vi "ZCR_IN_SIN_0_finder_temp.vi"(10 "Noise amplitude":dbl format="%.2p", 11 "ZCR IN":waveform(dbl)[](graph)) -> (3 "OFF SIN":i32[](array[numeric]))   [LabVIEW 2020, in "Library Commun.lvlib" / "Nodon_ZCR.lvclass"]
uses:
  Nodon_ZCR.lvclass
  <vilib>/Utility/miscctls.llb/LVRangeTypeDef.ctl
  Nodon_ZCR.lvclass/Nodon_ZCR.ctl
  <vilib>/measure/NI_MABase.lvlib
panel:
  out "Waveform Graph 3":waveform(dbl)[](graph)
  in  "Point 2":i32
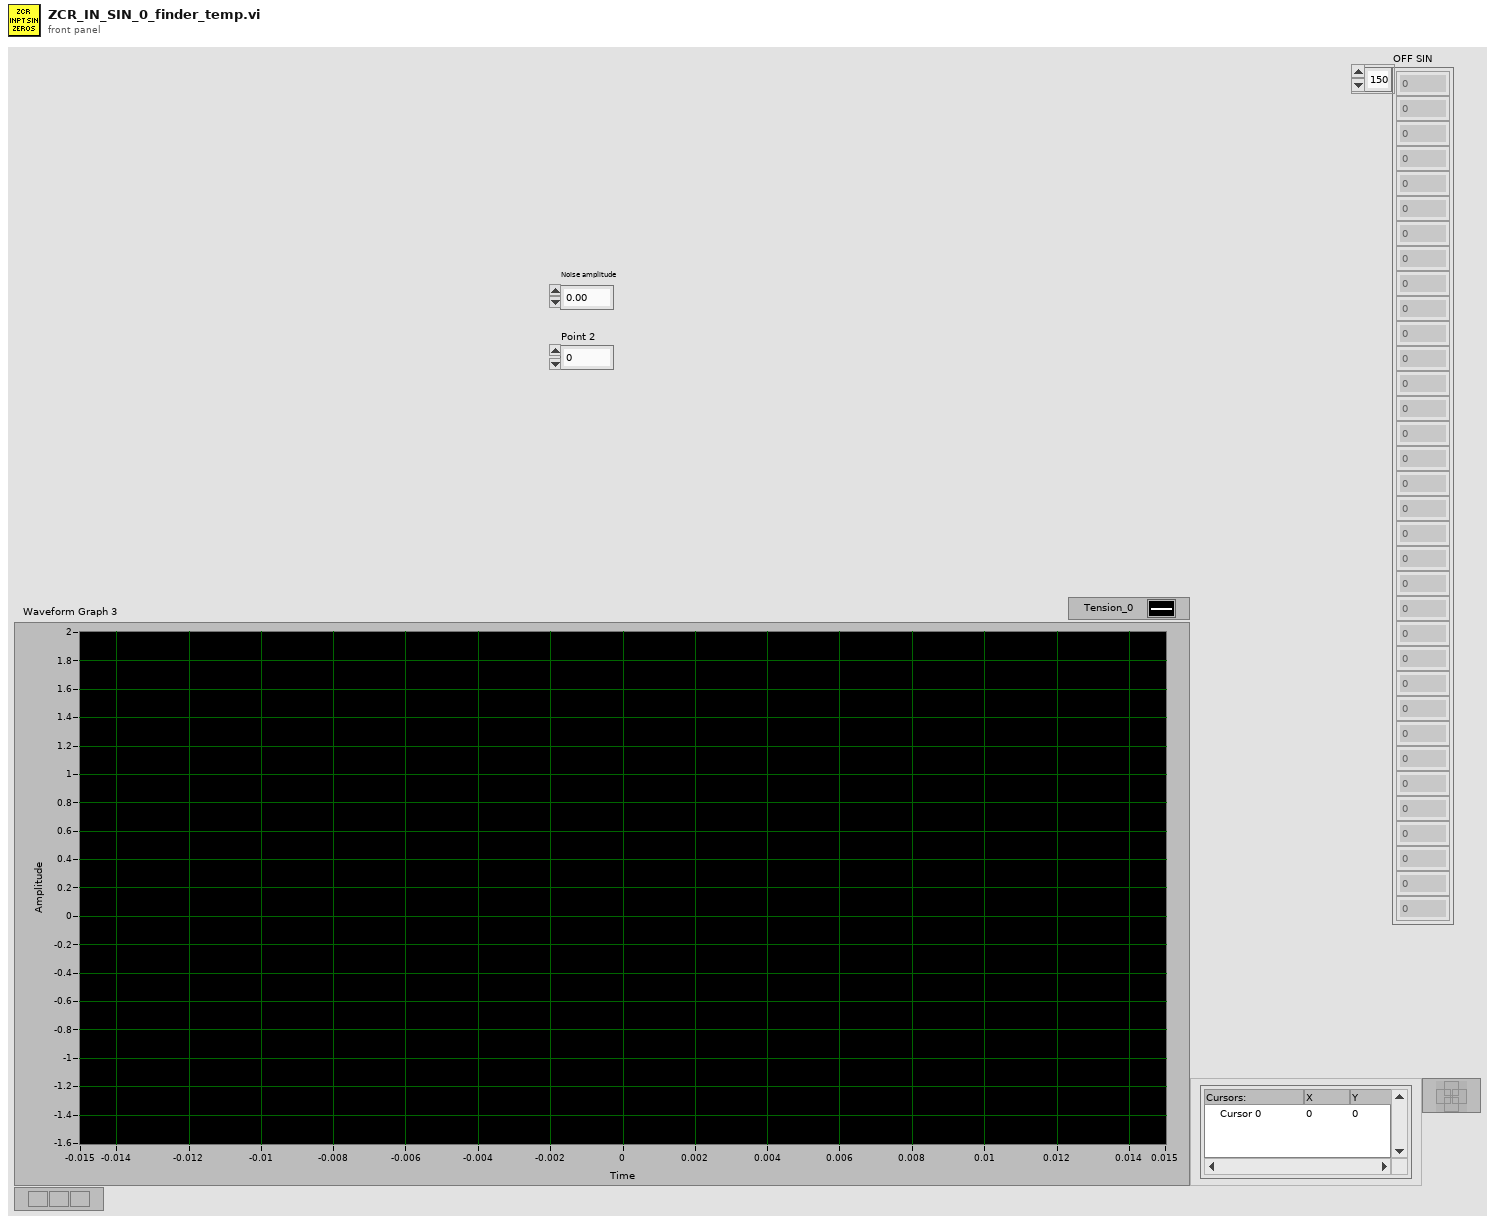
[diagram p1: front panel]
types:
  T1 = typedef "LVRangeTypeDef.ctl" = cluster{"Minimum":dbl, "Maximum":dbl, "Increment":dbl, "Minor Increment":dbl, "Start":dbl}
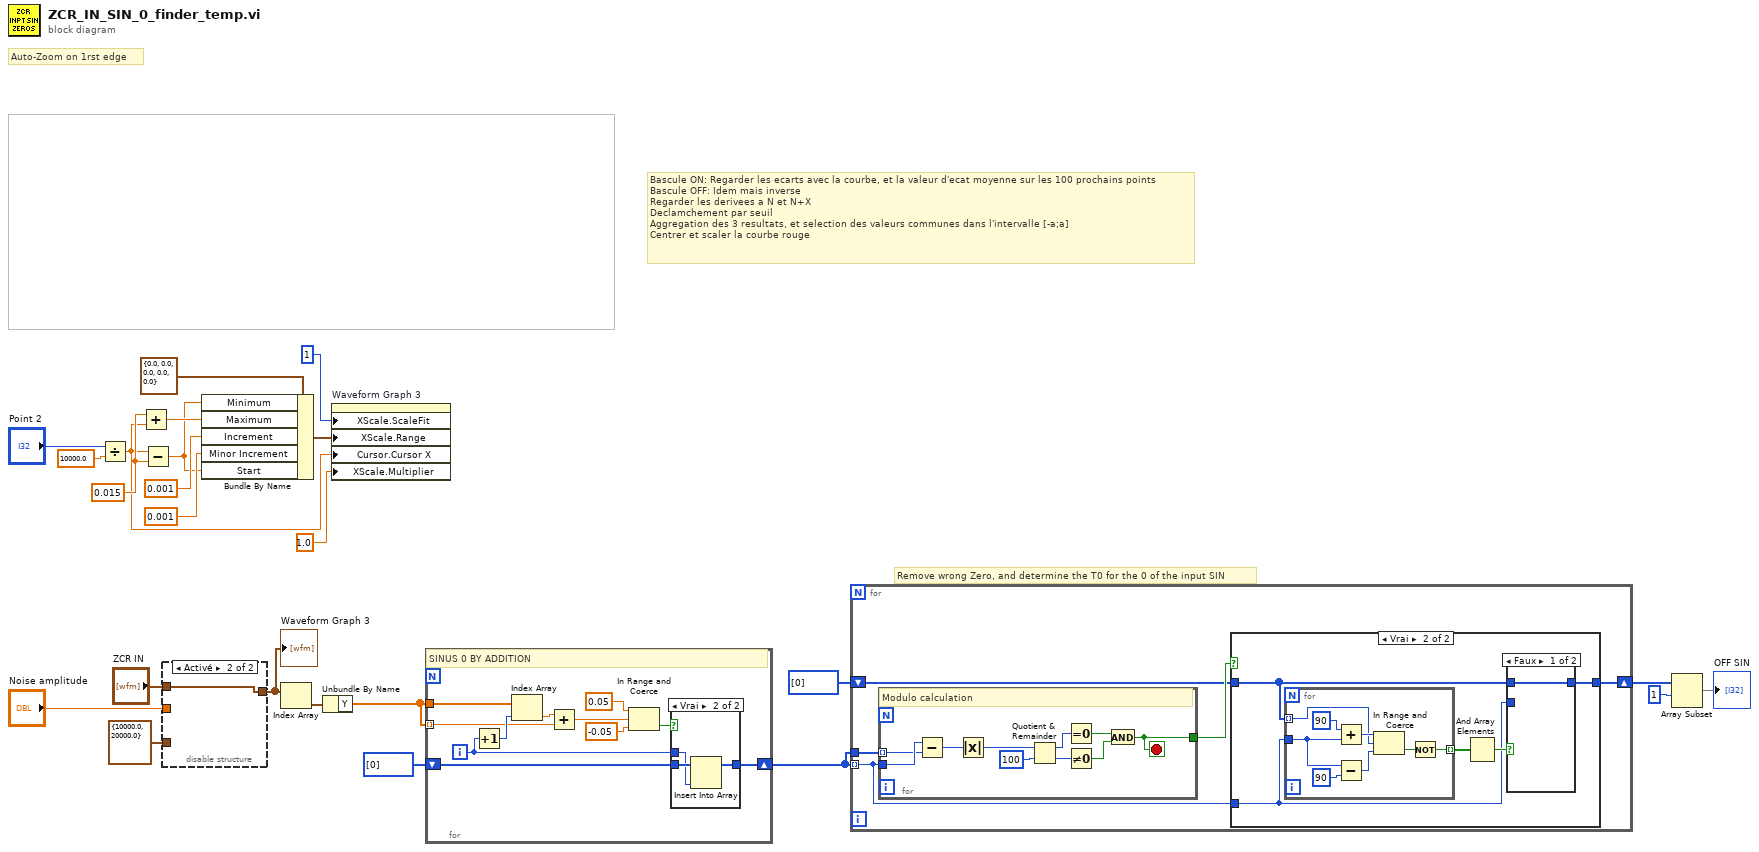
[diagram p0: block diagram]
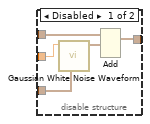
[diagram p2: hidden frame]
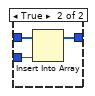
[diagram p4: hidden frame]
diagram:
  w20 = 0.015
  # "Bascule ON: Regarder les ecarts avec la courbe, et la valeur d'ecat moyenne sur les 100 prochains points\nBascule OFF: Idem mais inverse\nRegarder les derivees a N et N+X\nDeclamchement par seuil\nAggregation des 3 resultats, et selection des valeurs communes dans l'intervalle [-a;a]\nCentrer et scaler la courbe rouge"
  # "Remove wrong Zero, and determine the T0 for the 0 of the input SIN"
  # "Auto-Zoom on 1rst edge"
  n1 = Divide(x="Point 2", y=10000.0) -> (x/y=w11:dbl)
  n2 = Add(x=w20, y=w11) -> (x+y=w18:dbl)
  n3 = Subtract(x=w11, y=w20) -> (x-y=w15:dbl)
  n4 = disable-structure shown="Activé" {
    disable-tunnel: "Noise amplitude" -> [w29 _]
    disable-tunnel: cluster{"Fs":dbl, "#s":dbl} {"Fs"=10000.0, "#s"=20000.0} ("sampling info") -> [w28 _]
    disable-tunnel: [w26 w30] -> w9
    disable-tunnel: "ZCR IN" -> [w25 w30]
    frame Disabled {
      n5 = call <vilib>:"Gaussian White Noise Waveform.vi"("sampling info"=w28, "standard deviation"=w29) -> ("signal out"=w27:waveform(dbl))  [unwired: 8 in, 1 out]
      n6 = Add(1:w27, 2:w25) -> (0:w26:waveform(dbl)[])  [unwired: 1 in, 1 out]
    }
    frame Enabled {
    }
  }
  "Waveform Graph 3" <- w9
  n7 = Bundle By Name(cluster=T1 {"Minimum"=0.0, "Maximum"=0.0, "Increment"=0.0, "Minor Increment"=0.0, "Start"=0.0} ("X Scale.Range"), "Minimum"=w15, "Maximum"=w18, "Increment"=0.001, "Minor Increment"=0.001, "Start"=w15) -> (w14:T1)
  n8 = Index Array(array=w9) -> (element=w1:waveform(dbl))  [unwired: 1 in]
  n9 = Unbundle By Name(w1) -> ("Y"=w6:dbl[])
  n10 = property on="Waveform Graph 3" class="GraphWF (strict)"("XScale.ScaleFit"=u8 1 ("X Scale.Scale Fit"), "XScale.Range"=w14, "Cursor.Cursor X"=w11, "XScale.Multiplier"=1.0 ("X Scale.Offset and Multiplier:Multiplier")) -> ()  [unwired: 2 in, 2 out]
  n11 = for {
    tunnel: w6 -> [w41]
    tunnel: w6 -> [w38] mode=indexing
    shift-right: [w36] -> w8
    shift-left: i32[] [0] -> [w37]
    i -> [w35]
    # "SINUS 0 BY ADDITION"
    n12 = Increment(x=w35) -> (x+1=w40:i32)
    n13 = Index Array(array=w41, index=w40) -> (element=w39:dbl)
    n14 = Add(x=w39, y=w38) -> (x+y=w34:dbl)
    n15 = In Range and Coerce(upper limit=0.05 ("lower limit"), x=w34, lower limit=-0.05) -> (In Range?=w33:bool)  [unwired: 1 out]
    n16 = case shown="Vrai" w33 {
      tunnel: [w42 w44] -> w36
      tunnel: w37 -> [w42 w45]
      tunnel: w35 -> [_ w43]
      frame False {
      }
      frame True {
        n17 = Insert Into Array(array=w45, new element=w43) -> (w44:i32[])  [unwired: 1 in]
      }
    }
  }
  n18 = for {
    tunnel: w8 -> [w46] mode=indexing
    tunnel: w8 -> [w50]
    shift-right: [w47] -> w5
    shift-left: i32[] [0] -> [w48]
    n19 = for {
      tunnel: w46 -> [w78]
      tunnel: w50 -> [w77] mode=indexing
      tunnel: [w69] -> w49
      stop <- w69 stop-if-true
      # "Modulo calculation"
      n20 = Subtract(x=w78, y=w77) -> (x-y=w76:i32)
      n21 = Absolute Value(x=w76) -> (abs(x)=w75:i32)
      n22 = Quotient & Remainder(x=w75, y=100) -> (x-y*floor(x/y)=w73:i32, floor(x/y)=w72:i32)
      n23 = Equal To 0?(x=w73) -> (x = 0?=w71:bool)
      n24 = Not Equal To 0?(x=w72) -> (x != 0?=w70:bool)
      n25 = And(x=w71, y=w70) -> (x .and. y?=w69:bool)
    }
    n26 = case shown="Vrai" w49 {
      tunnel: w48 -> [w51 w54]
      tunnel: [w51 w53] -> w47
      tunnel: w46 -> [_ w52]
      frame False {
      }
      frame True {
        n27 = for {
          tunnel: w52 -> [w64]
          tunnel: w54 -> [w61] mode=indexing
          tunnel: [w62] -> w56 mode=indexing
          n28 = Add(x=90, y=w64) -> (x+y=w66:i32)
          n29 = Subtract(x=w64, y=90) -> (x-y=w65:i32)
          n30 = In Range and Coerce(upper limit=w66, x=w61, lower limit=w65) -> (In Range?=w63:bool)  [unwired: 1 out]
          n31 = Not(x=w63) -> (.not. x?=w62:bool)
        }
        n32 = And Array Elements(Boolean array=w56) -> (logical AND=w55:bool)
        n33 = case shown="Faux" w55 {
          tunnel: w54 -> [w57 w59]
          tunnel: [w57 w60] -> w53
          tunnel: w52 -> [_ w58]
          frame False {
          }
          frame True {
            n34 = Insert Into Array(array=w59, new element=w58) -> (w60:i32[])  [unwired: 1 in]
          }
        }
      }
    }
  }
  n35 = Array Subset(array=w5, index=1) -> (→"OFF SIN":i32[])  [unwired: 1 in]
